vi "Center_Prompt.vi"(0 "Data Cluster":T1 {"Shaft"."dmin" format="%#_7g"; "Shaft"."dmax" format="%#_7g"; "Shaft"."Fundamental Dev" format="%#_7g"; "Shaft"."Tolerance Grade (IT) Shaft" format="%#_7g"; "Hole"."Dmin" format="%#_7g"; "Hole"."Tolerance Grade (IT)" format="%#_7g"}, 2 "Alignment":T6={"Horizontal"=enum."Center", "Vertical"=enum."Center"} caption="Alignment (Center, Center)", 3 "Ref VI":refnum<vi>, 5 "Error In":errorcluster) -> (6 "Data Cluster Out":T1 {"Shaft"."dmin" format="%#_7g"; "Shaft"."dmax" format="%#_7g"; "Shaft"."Fundamental Dev" format="%#_7g"; "Shaft"."Tolerance Grade (IT) Shaft" format="%#_7g"; "Hole"."Dmin" format="%#_7g"; "Hole"."Tolerance Grade (IT)" format="%#_7g"}, 8 "error out":errorcluster)   [LabVIEW 2023]
uses:
  <vilib>/MGI/Panel Manager/Panel/Window Position/Reference Position/Alignment.ctl
  <vilib>/MGI/Panel Manager/Panel/Window Position/Reference Position/Horizontal Alignment.ctl
  <vilib>/MGI/Panel Manager/Panel/Window Position/Reference Position/Vertical Alignment.ctl
  TypeDef/Data_Cluster.ctl
  <vilib>/MGI/Panel Manager/Panel/Panel/Window/Window.lvclass
  TypeDef/Units.ctl
  TypeDef/Method_Info.ctl
  TypeDef/Hole_Data.ctl
  TypeDef/Shaft_Data.ctl
  <vilib>/MGI/Panel Manager/Panel/Window Position/Reference Position/Offset/Absolute Offset/Absolute Offset.lvclass
  C:/Program Files (x86)/National Instruments/LabVIEW 2023/vi.lib/MGI/Panel Manager/Panel/Window Position/Reference Position/Offset/Offset.lvclass
  <vilib>/MGI/Panel Manager/Panel/Window Position/Reference Position/Ref VI/Ref VI.lvclass
  C:/Program Files (x86)/National Instruments/LabVIEW 2023/vi.lib/MGI/Panel Manager/Panel/Window Position/Window Position.lvclass
  <vilib>/MGI/Panel Manager/Panel/Window Position/Reference Position/Offset/Absolute Offset/No Offset.vi
  <vilib>/MGI/Panel Manager/Panel/Window Position/Reference Position/Ref VI/Ref VI.vi
  <vilib>/MGI/Panel Manager/Panel/Panel/Window/Window.vi
  <vilib>/MGI/Panel Manager/Panel/Panel.lvlib
  C:/Program Files (x86)/National Instruments/LabVIEW 2023/vi.lib/MGI/Panel Manager/Panel/Window Position/Reference Position/Offset/Absolute Offset/Absolute Offset.lvclass
  C:/Program Files (x86)/National Instruments/LabVIEW 2023/vi.lib/MGI/Panel Manager/Panel/Window Position/Reference Position/Reference Position.lvclass
  C:/Program Files (x86)/National Instruments/LabVIEW 2023/vi.lib/MGI/Panel Manager/Panel/Window Position/Reference Position/Ref VI/Ref VI.lvclass
  <vilib>/MGI/Panel Manager/Panel/Window Position/Reference Position/Reference Position.lvclass
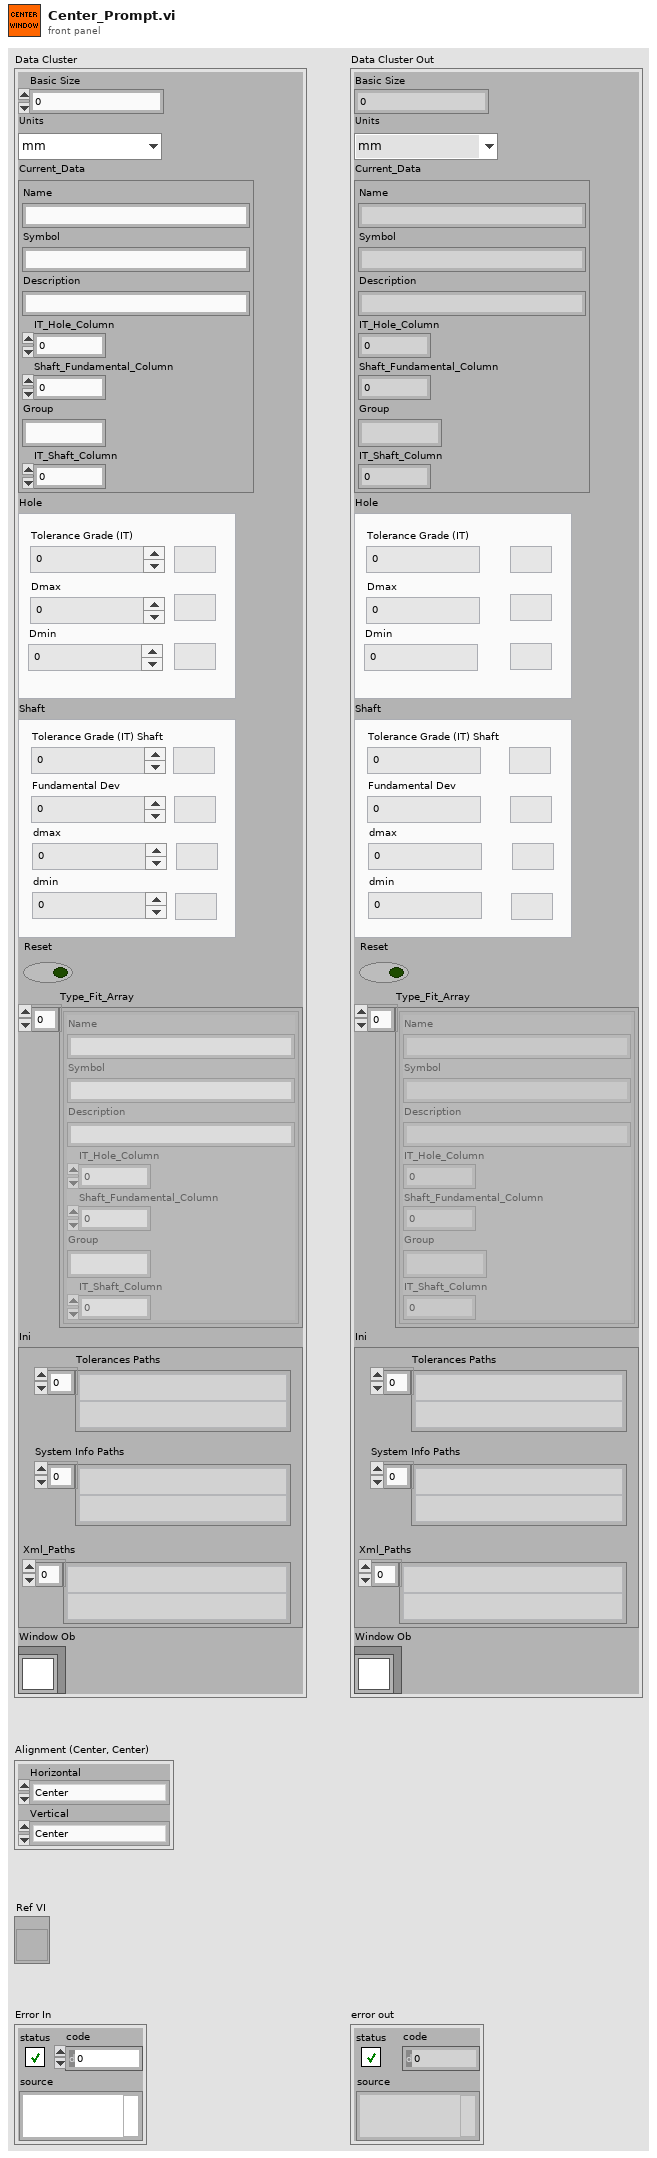
[diagram p1: front panel]
types:
  T1 = typedef "Data_Cluster.ctl" = cluster{"Basic Size ":dbl, "Units":T2, "Current_Data":T3, "Hole":T4, "Shaft":T5, "Reset":bool, "Type_Fit_Array":T3[], "Ini":cluster{"Tolerances Paths":path[], "System Info Paths":path[], "Xml_Paths":path[]}, "Window Ob":refnum<class "Window.lvclass">}
  T2 = typedef "Units.ctl" = enum16{"mm", "in"}
  T3 = typedef "Method_Info.ctl" = cluster{"Name":string, "Symbol":string, "Description":string, "IT_Hole_Column":i32, "Shaft_Fundamental_Column":i32, "Group":string, "IT_Shaft_Column":i32}
  T4 = typedef "Hole_Data.ctl" = cluster{"Tolerance Grade (IT)":dbl, "Dmax":dbl, "Units Hole":cluster{"units_it":string, "units_Dmax\nUnits_Dmax":string, "Units_Dmin":string}, "Dmin":dbl}
  T5 = typedef "Shaft_Data.ctl" = cluster{"Tolerance Grade (IT) Shaft":dbl, "Units Shaft":cluster{"Units_FundamentalDev":string, "Units_dmax":string, "Units_dmin":string, "Units_IT_Shaft":string}, "Fundamental Dev":dbl, "dmax":dbl, "dmin":dbl}
  T6 = typedef "Panel.lvlib/Reference Position.lvclass/Alignment.ctl" = cluster{"Horizontal":T7, "Vertical":T8}
  T7 = typedef "Panel.lvlib/Reference Position.lvclass/Horizontal Alignment.ctl" = enum16{"Left", "Center", "Right"}
  T8 = typedef "Panel.lvlib/Reference Position.lvclass/Vertical Alignment.ctl" = enum16{"Top", "Center", "Bottom"}
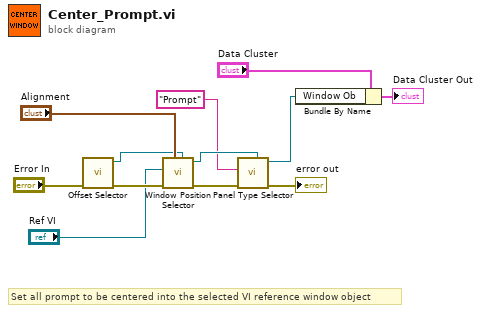
[diagram p0: block diagram]
diagram:
  # "Set all prompt to be centered into the selected VI reference window object"
  n1 = call-poly <vilib>:"Offset Selector.vi"("Error In"="Error In") -> ("Error Out"=w10:errorcluster, "Absolute Offset Out"=w9:refnum<class "Absolute Offset.lvclass">)  [unwired: 9 in]
  n2 = call-poly <vilib>:"Window Position Selector.vi"("Offset"=w9, "Alignment"="Alignment", "Error In"=w10, "Ref VI"="Ref VI") -> ("Error Out"=w7:errorcluster, "Ref VI out"=w6:refnum<class "Ref VI.lvclass">)  [unwired: 6 in]
  n3 = call-poly <vilib>:"Panel Type Selector.vi"("Window Position"=w6, "error in (no error)"=w7, "Default Title"="Prompt") -> ("error out"=→"error out":errorcluster, "Window out"=w1:refnum<class "Window.lvclass">)  [unwired: 7 in]
  n4 = Bundle By Name(cluster="Data Cluster", "Window Ob"=w1) -> (→"Data Cluster Out":T1)
